vi "Check Package.vi"(8 "error in (no error)":errorcluster, 10 "Package":refnum<class "PackageAbstract.lvclass">, 11 "SyncAction in":refnum<class "SyncAction.lvclass">) -> (0 "error out":errorcluster, 2 "Problems":string[](array[string]), 3 "SyncAction out":refnum<class "SyncAction.lvclass">)   [LabVIEW 2020, in "GPackTools.lvlib" / "SyncAction.lvclass"]
uses:
  SyncAction.lvclass
  GPack/PackageAbstract/PackageAbstract.lvclass
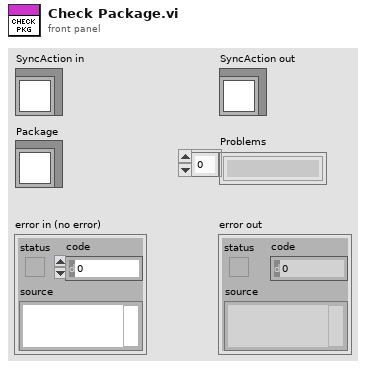
[diagram p1: front panel]
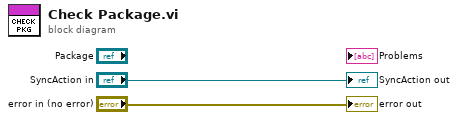
[diagram p0: block diagram]
diagram:
  "error out" <- "error in (no error)"
  "SyncAction out" <- "SyncAction in"
